vi "Main.vi"(8 "error in":errorcluster, 11 "Message Pump":refnum<class "Message Pump.lvclass">) -> (0 "error out":errorcluster, 3 "Message Pump out":refnum<class "Message Pump.lvclass">)   [LabVIEW 2023, in "Abstract Hardware.lvlib" / "Message Pump.lvclass"]
doc: "The <b>Queued Message Handler</b> of the Worker that owns this VI."
uses:
  Message Pump.lvclass
  Initialization Data.ctl
  Response Cases.ctl
  <vilib>/addons/_Workers/Library/Case Label.ctl
  Message Pump.lvclass/Message Pump.ctl
  rqp_Set EHL Timeout.ctl
  <vilib>/Utility/error.llb/Error Cluster From Error Code.vi
  <vilib>/ErrorRing/Error Ring.xnode
  <vilib>/addons/_Workers/Library/Workers.lvlib
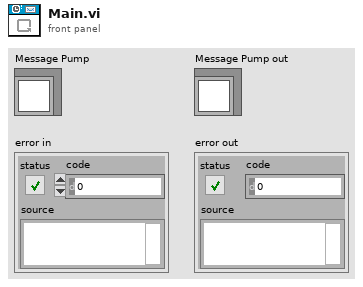
[diagram p1: front panel]
types:
  T1 = typedef "Abstract Hardware.lvlib/Message Pump.lvclass/Initialization Data.ctl" = cluster{"Response Cases":T2}
  T2 = typedef "Abstract Hardware.lvlib/Message Pump.lvclass/Response Cases.ctl" = cluster{"Timer Elapsed":T3}
  T3 = typedef "Workers.lvlib/Case Label.ctl" = string
  T4 = typedef "Abstract Hardware.lvlib/Message Pump.lvclass/rqp_Set EHL Timeout.ctl" = cluster{"Timeout (ms)":i32}
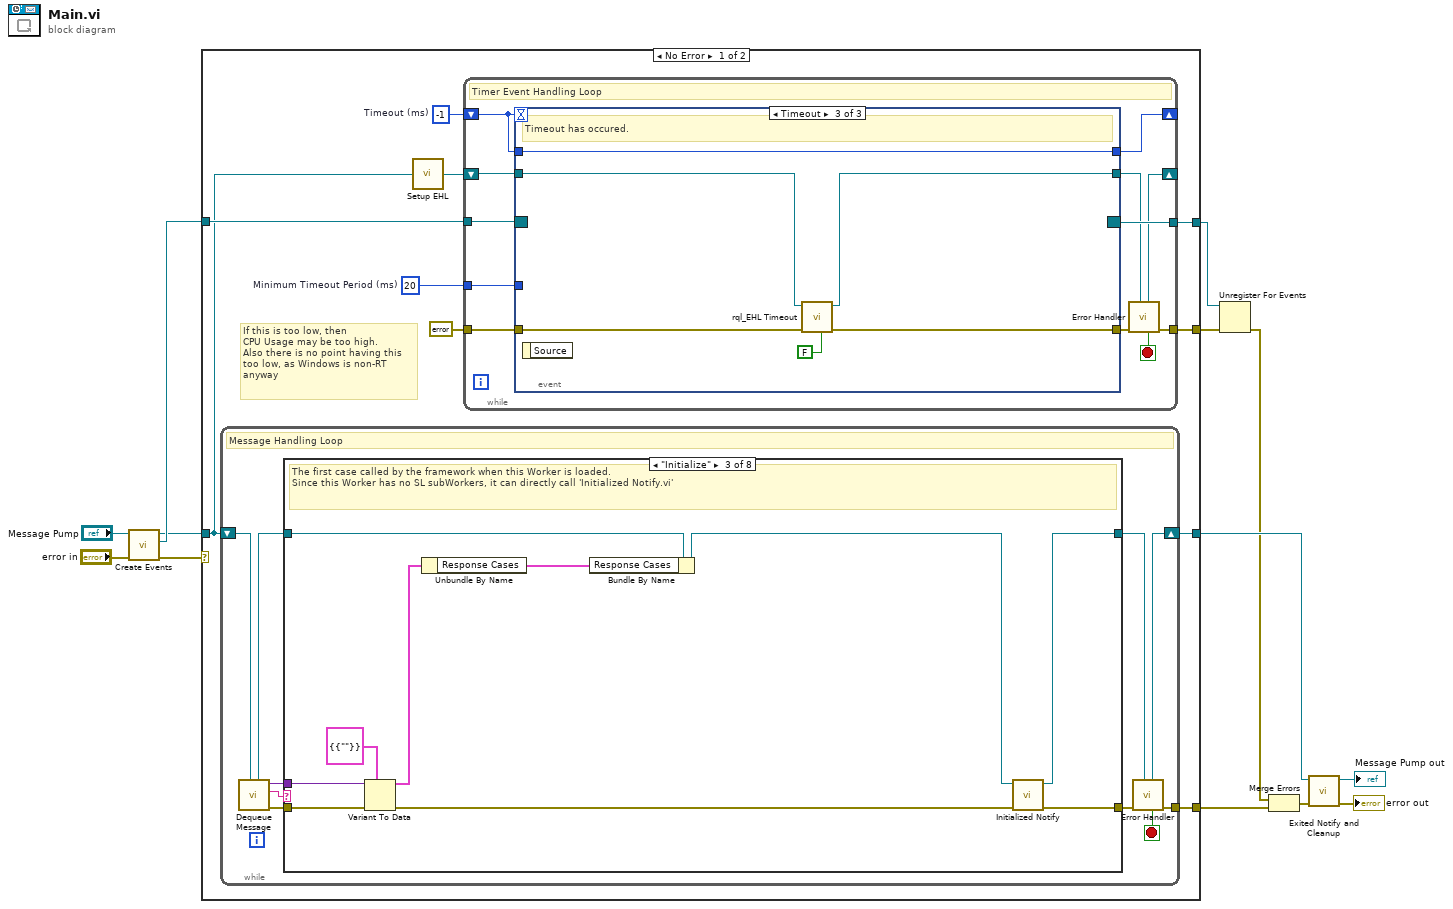
[diagram p0: block diagram]
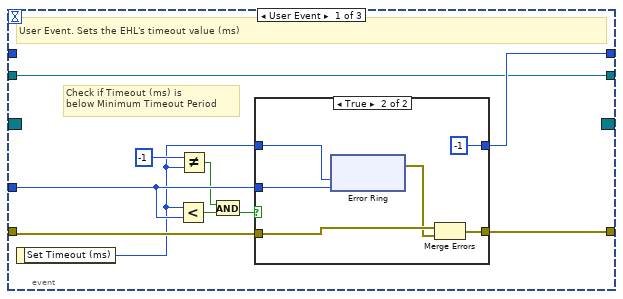
[diagram p2: hidden frame]
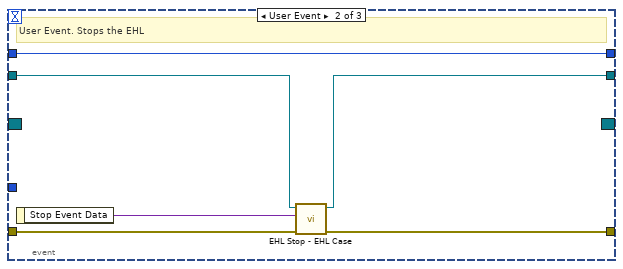
[diagram p4: hidden frame]
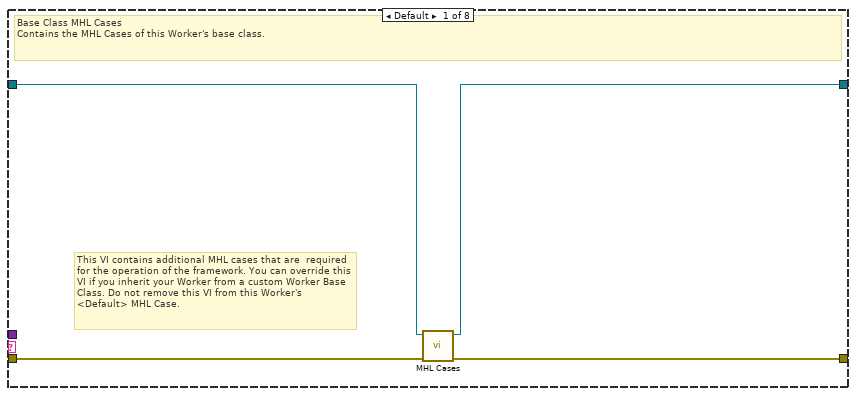
[diagram p5: hidden frame]
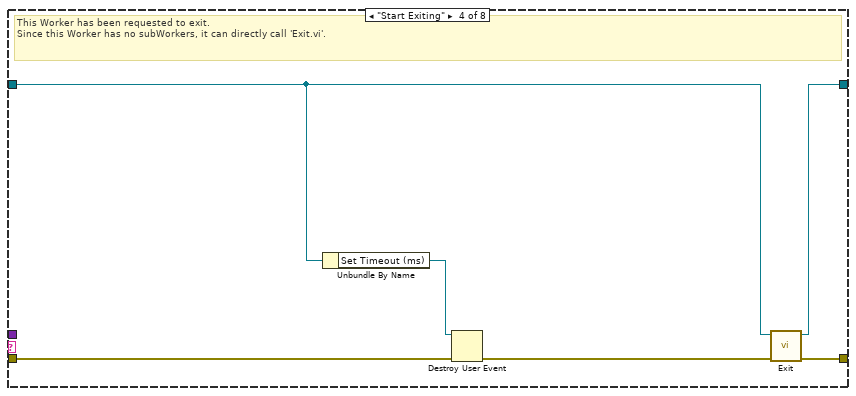
[diagram p7: hidden frame]
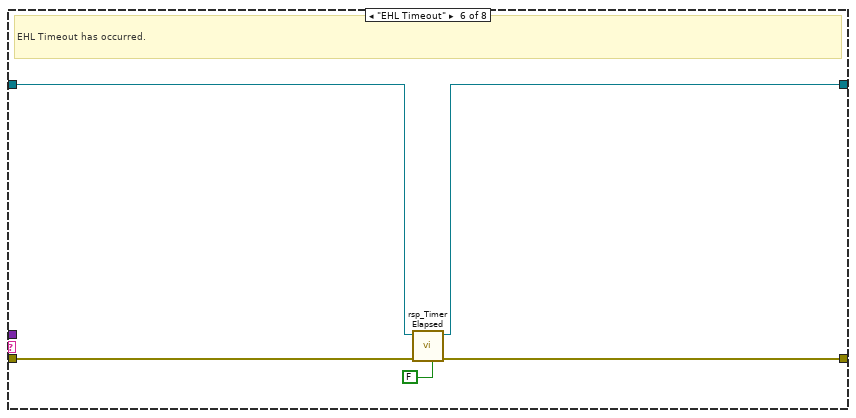
[diagram p9: hidden frame]
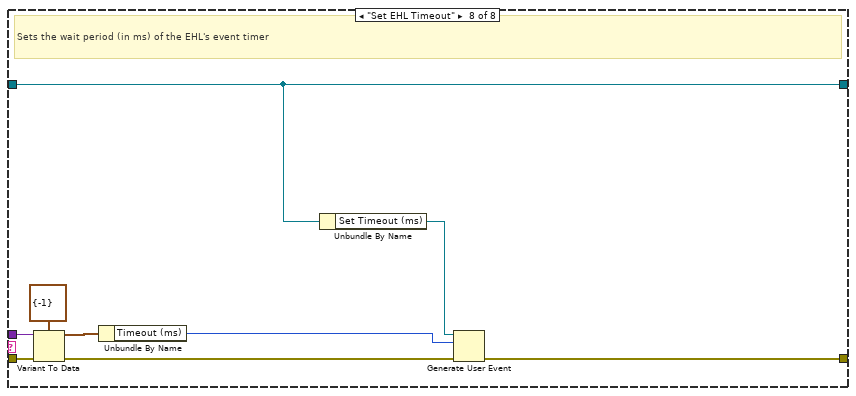
[diagram p11: hidden frame]
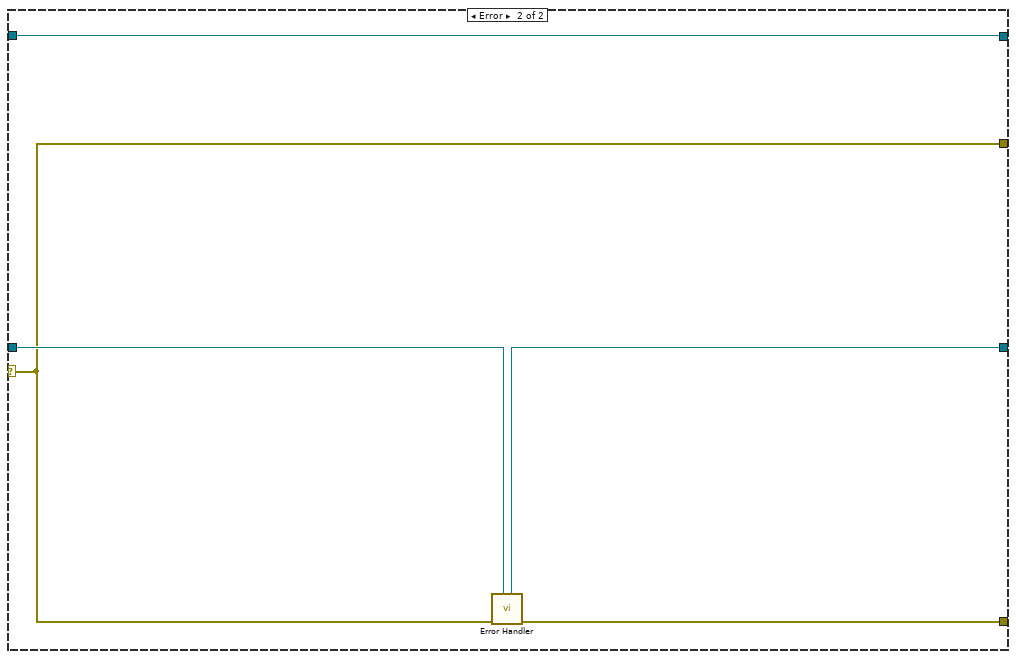
[diagram p12: hidden frame]
diagram:
  n1 = call "Create Events.vi"("error in"="error in", "Message Pump in"="Message Pump") -> ("error out"=w8:errorcluster, "Event Registration Refnum"=w9:refnum<event-registration>, "Message Pump out"=w4:refnum<class "Message Pump.lvclass">)  [unwired: 6 in]
  n2 = case shown="No Error" w8 {
    tunnel: w4 -> [w15 w127]
    tunnel: [w23 w128] -> w12
    tunnel: [w22 w126] -> w13
    selector: w8 -> [_ w125]
    tunnel: [w16 w125] -> w2
    tunnel: [w18 w124] -> w3
    tunnel: w9 -> [w17 w124]
    frame No Error {
      w21 = 20  # Minimum Timeout Period (ms)
      w20 = -1  # Timeout (ms)
      # "If this is too low, then \nCPU Usage may be too high.\nAlso there is no point having this\ntoo low, as Windows is non-RT\nanyway"
      n3 = while {
        shift-right: [w81] -> w22
        shift-left: w15 -> [w83]
        tunnel: [w82] -> w23
        stop <- w75 stop-if-true
        # "Message Handling Loop"
        n4 = call-dynamic "Dequeue Message.vi"("Worker"=w83) -> ("error out"=w80:errorcluster, "Case out"=w76:string, "Data out"=w74:variant, "Worker out"=w78:refnum<class "Message Pump.lvclass">)  [unwired: 6 in, 1 out]
        n5 = case "WORKERS MHL Case Structure (DO NOT CHANGE LABEL NAME)" shown="\"Initialize\"" w76 {
          tunnel: w80 -> [w87 w88 w97 w101 w107 w112 w114 w123]
          tunnel: [w86 w88 w99 w105 w107 w111 w114 w115] -> w79
          tunnel: w78 -> [w85 w89 w92 w100 w106 w110 w113 w117]
          tunnel: [w84 w89 w98 w104 w106 w109 w113 w117] -> w77
          tunnel: w74 -> [_ _ w96 _ _ _ _ w121]
          frame Default {
            # "This VI contains additional MHL cases that are  required for the operation of the framework. You can override this VI if you inherit your Worker from a custom Worker Base Class. Do not remove this VI from this Worker's <Default> MHL Case."
            # "Base Class MHL Cases\nContains the MHL Cases of this Worker's base class."
            n6 = call-dynamic "MHL Cases.vi"("error in"=w87, "Worker in"=w85) -> ("error out"=w86:errorcluster, "Worker out"=w84:refnum<class "Message Pump.lvclass">)  [unwired: 8 in]
          }
          frame "------------ FRAMEWORK CASES -----------" {
            # "Start of Workers Framework Cases"
          }
          frame "Initialize" {
            # "The first case called by the framework when this Worker is loaded.\nSince this Worker has no SL subWorkers, it can directly call 'Initialized Notify.vi'"
            n7 = Variant To Data(error in=w97, type=T1 {"Response Cases"={"Timer Elapsed"=""}} ("Initialize Data"), Variant=w96) -> (data=w94:T1, error out=w93:errorcluster)
            n8 = Unbundle By Name(w94) -> ("Response Cases"=w90:T2)
            n9 = Bundle By Name(cluster=w92, "Response Cases"=w90) -> (w91:refnum<class "Message Pump.lvclass">)
            n10 = call-dynamic "Initialized Notify.vi"("error in"=w93, "Worker"=w91) -> ("error out"=w99:errorcluster, "dup Worker out"=w98:refnum<class "Message Pump.lvclass">)  [unwired: 8 in]
          }
          frame "Start Exiting" {
            # "This Worker has been requested to exit.\nSince this Worker has no subWorkers, it can directly call 'Exit.vi'."
            n11 = Unbundle By Name(w100) -> ("Set Timeout (ms)"=w102:refnum<user-event>)
            n12 = Destroy User Event(user event=w102, error in=w101) -> (error out=w103:errorcluster)
            n13 = call-dynamic "Exit.vi"("error_in"=w103, "Worker"=w100) -> ("error out"=w105:errorcluster, "dup Worker out"=w104:refnum<class "Message Pump.lvclass">)  [unwired: 8 in]
          }
          frame "------------- LOCAL API CASES -------------" {
            # "Start of Workers Local API Cases"
          }
          frame "EHL Timeout" {
            # "EHL Timeout has occurred."
            n14 = call "rsp_Timer Elapsed.vi"("Show in Debugger?"=FALSE, "error in"=w112, "Message Pump in"=w110) -> ("error out"=w111:errorcluster, "dup Message Pump out"=w109:refnum<class "Message Pump.lvclass">)  [unwired: 7 in]
          }
          frame "------------- PUBLIC API CASES -------------" {
            # "Start of Workers Public API Cases"
          }
          frame "Set EHL Timeout" {
            # "Sets the wait period (in ms) of the EHL's event timer"
            n15 = Variant To Data(error in=w123, type=T4 {"Timeout (ms)"=-1} ("Data"), Variant=w121) -> (data=w120:T4, error out=w118:errorcluster)
            n16 = Unbundle By Name(w120) -> ("Timeout (ms)"=w116:i32)
            n17 = Unbundle By Name(w117) -> ("Set Timeout (ms)"=w119:refnum<user-event>)
            n18 = Generate User Event(user event=w119, event data cluster=w116, error in=w118) -> (error out=w115:errorcluster)  [unwired: 1 in, 1 out]
          }
        }
        n19 = call-dynamic "Error Handler.vi"("Worker"=w77, "error_in"=w79) -> ("error out"=w82:errorcluster, "Stop Loop"=w75:bool, "Worker out"=w81:refnum<class "Message Pump.lvclass">)  [unwired: 7 in]
      }
      n20 = call-dynamic "Setup EHL.vi"("Worker"=w15) -> ("Worker out"=w14:refnum<class "Message Pump.lvclass">)  [unwired: 14 in]
      n21 = while "Event Handling Loop" {
        shift-right: [w24] -> _
        shift-left: w20 -> [w34]
        tunnel: errorcluster {"status"=FALSE, "code"=0, "source"=""} ("error IO") -> [w35]
        tunnel: [w29] -> w16
        tunnel: w17 -> [w33]
        tunnel: [w32] -> w18
        tunnel: w21 -> [w31]
        shift-right: [w26] -> _
        shift-left: w14 -> [w28]
        stop <- w25 stop-if-true
        # "Timer Event Handling Loop"
        n22 = event shown="[2] Timeout" {
          selector: w33 -> [_ _ _]
          dyn-events: [_ _ _] -> w32
          timeout: w34 -> [_ _ _]
          tunnel: w35 -> [w43 w67 w73]
          tunnel: [w44 w65 w71] -> w30
          tunnel: w34 -> [_ w66 w72]
          tunnel: [w41 w66 w72] -> w24
          tunnel: w31 -> [w42 _ _]
          tunnel: w28 -> [w36 w64 w70]
          tunnel: [w36 w63 w69] -> w27
          event User Event {
            # "Check if Timeout (ms) is\nbelow Minimum Timeout Period"
            # "User Event. Sets the EHL's timeout value (ms)"
            n23 = event-data() -> ("Set Timeout (ms)"=w38:i32)  [unwired: 1 in]
            n24 = Less?(x=w38, y=w42) -> (x < y?=w45:bool)
            n25 = Not Equal?(x=-1 ("Set Timeout (ms)"), y=w38) -> (x != y?=w37:bool)
            n26 = And(x=w37, y=w45) -> (x .and. y?=w40:bool)
            n27 = case shown="True" w40 {
              tunnel: [w47 w51] -> w44
              tunnel: w43 -> [w47 w52]
              tunnel: w38 -> [w46 w49]
              tunnel: w42 -> [_ w48]
              tunnel: [w46 -1 ("Set Timeout (ms)")] -> w41
              frame False {
              }
              frame True {
                n28 = xnode "Error Ring"("parameter 0"=w49, "parameter 1"=w48) -> ("error out"=w50:errorcluster)
                n29 = Merge Errors(w52, w50) -> (w51:errorcluster)
              }
            }
          }
          event User Event {
            # "User Event. Stops the EHL"
            n30 = event-data() -> ("Stop Event Data"=w62:variant)  [unwired: 1 in]
            n31 = call-dynamic "EHL Stop - EHL Case.vi"("error in"=w67, "Stop Event Data"=w62, "Worker"=w64) -> ("error out"=w65:errorcluster, "Worker out"=w63:refnum<class "Message Pump.lvclass">)  [unwired: 7 in]
          }
          event Timeout {
            # "Timeout has occured."
            n32 = event-data() -> ()  [unwired: 1 in, 1 out]
            n33 = call "rql_EHL Timeout.vi"("Show in Debugger?"=FALSE, "error in"=w73, "Message Pump in"=w70) -> ("error out"=w71:errorcluster, "dup Message Pump out"=w69:refnum<class "Message Pump.lvclass">)  [unwired: 7 in]
          }
        }
        n34 = call-dynamic "Error Handler.vi"("Worker"=w27, "error_in"=w30) -> ("error out"=w29:errorcluster, "Stop Loop"=w25:bool, "Worker out"=w26:refnum<class "Message Pump.lvclass">)  [unwired: 7 in]
      }
    }
    frame Error {
      n35 = call-dynamic "Error Handler.vi"("Worker"=w127, "error_in"=w125) -> ("error out"=w128:errorcluster, "Worker out"=w126:refnum<class "Message Pump.lvclass">)  [unwired: 7 in, 1 out]
    }
  }
  n36 = Unregister For Events(event registration refnum=w3, error in=w2) -> (error out=w1:errorcluster)
  n37 = Merge Errors(w1, w12) -> (w11:errorcluster)
  n38 = call-dynamic "Exited Notify and Cleanup.vi"("error_in"=w11, "Worker"=w13) -> ("error out"=→"error out":errorcluster, "dup Worker out"=→"Message Pump out":refnum<class "Message Pump.lvclass">)  [unwired: 8 in]
